vi "SetTilesLoopDeltaT.vi"(11 "TilesLoopData in":T1) -> (3 "TilesLoopData out":T1)   [LabVIEW 2019, in "RT_Game.lvlib" / "Engine.lvclass"]
uses:
  Engine.lvclass
  TilesLoopData.ctl
  Coordinate.ctl
  SlideJob.ctl
  ScreenSide.ctl
  FPGA_Interface.ctl
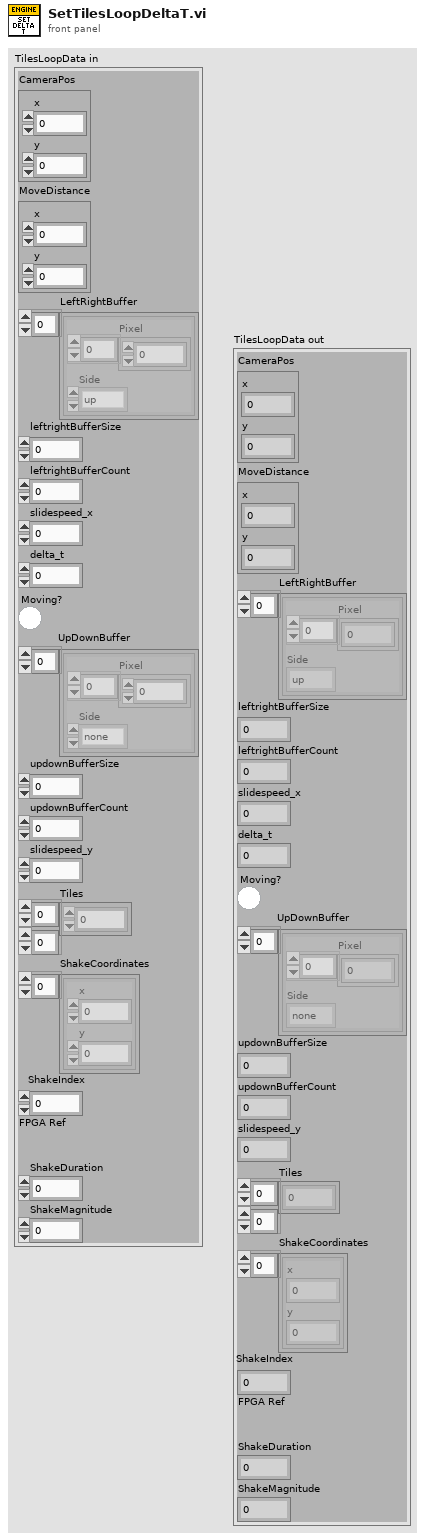
[diagram p1: front panel]
types:
  T1 = typedef "RT_Game.lvlib/Engine.lvclass/TilesLoopData.ctl" = cluster{"CameraPos":T2, "MoveDistance":T2, "LeftRightBuffer":T3[], "leftrightBufferSize":i16, "leftrightBufferCount":i16, "slidespeed_x":dbl, "delta_t":dbl, "Moving?":bool, "UpDownBuffer":T3[], "updownBufferSize":i16, "updownBufferCount":i16, "slidespeed_y":dbl, "Tiles":u32[][], "ShakeCoordinates":T2[], "ShakeIndex":i16, "FPGA Ref":T5, "ShakeDuration":dbl, "ShakeMagnitude":dbl}
  T2 = typedef "RT_Game.lvlib/Engine.lvclass/Coordinate.ctl" = cluster{"x":dbl, "y":dbl}
  T3 = typedef "RT_Game.lvlib/Engine.lvclass/SlideJob.ctl" = cluster{"Pixel":u32[], "Side":T4}
  T4 = typedef "RT_Game.lvlib/Engine.lvclass/ScreenSide.ctl" = enum16{"up", "down", "left", "right", "none"}
  T5 = typedef "FPGA_Interface.ctl" = refnum<k20>
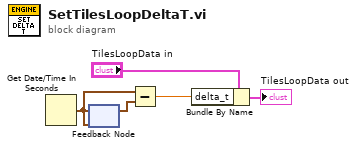
[diagram p0: block diagram]
diagram:
  n1 = Get Date/Time In Seconds() -> (seconds since 1Jan1904=w3:timestamp)
  n2 = feedback-in #1(w3) -> ()
  n3 = feedback #1(w3) -> (w2:timestamp)
  n4 = Subtract(x=w3, y=w2) -> (x-y=w1:dbl)
  n5 = Bundle By Name(cluster="TilesLoopData in", "delta_t"=w1) -> (→"TilesLoopData out":T1)
